vi "FTW-XML-Construct.vi"(5 "XML String":string, 11 "error in":errorcluster) -> (4 "XML Document":refnum<k20>, 15 "error out":errorcluster)   [LabVIEW 2013, in "XML.lvlib"]
uses:
  XML.lvlib
  DOMDefRefCommand.ctl
  <resource>/objmgr/DOMUserDefRef.rc
panel:
  # "Inputs"
  # "Outputs"
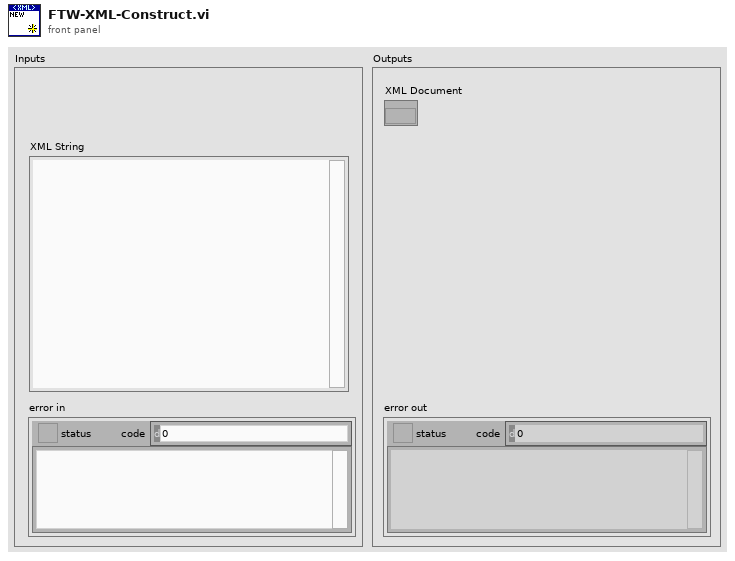
[diagram p1: front panel]
types:
  T1 = typedef "DOMDefRefCommand.ctl" = enum16{"No Command - Error", "Initialise", "Open Document", "Allocate RefNum", "Close Document"}
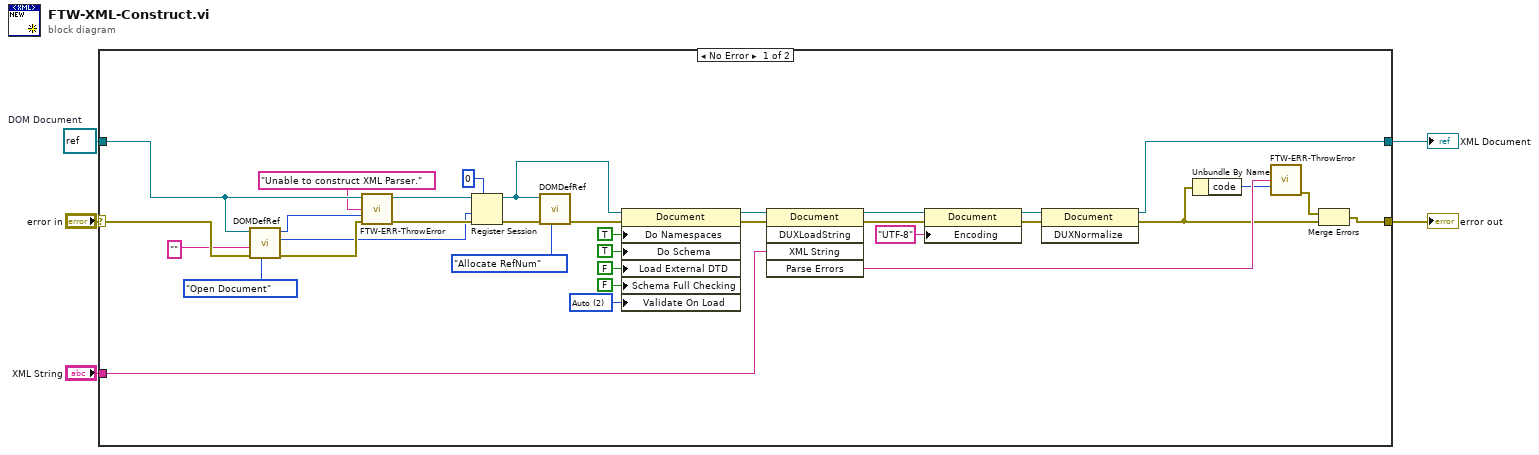
[diagram p0: block diagram]
diagram:
  w1 = refnum<k20> refnum  # DOM Document
  n1 = case shown="No Error" "error in" {
    selector: "error in" -> [w38 w40]
    tunnel: [w26 w40] -> w5
    tunnel: [w18 w39] -> w3
    tunnel: "XML String" -> [w30 _]
    tunnel: w1 -> [w25 w39]
    frame No Error {
      w33 = 2 items=["Never", "Always", "Auto"] ("Validate On Load")
      n2 = call "DOMDefRef.vi"("DOMUserDefRefCommand"=DOMDefRefCommand."Open Document", "error in (no error)"=w38, "Name"="", "Refnum in"=w25) -> ("error out"=w24:errorcluster, "Document Session"=w20:u64, "Return"=w21:i32)  [unwired: 2 in]
      n3 = call "FTW-ERR-ThrowError.vi"("Error Message"="Unable to construct XML Parser.", "Error Code"=w21, "error in"=w24) -> ("error out"=w23:errorcluster)  [unwired: 12 in]
      n4 = Register Session(7:0 ("cleanup mode (default to class = 0)"), 8:w23, 9:w20, 11:w25) -> (0:w9:errorcluster, 3:w8:refnum<k20>)  [unwired: 1 in]
      n5 = call "DOMDefRef.vi"("DOMUserDefRefCommand"=DOMDefRefCommand."Allocate RefNum", "error in (no error)"=w9, "Refnum in"=w8) -> ("error out"=w6:errorcluster)  [unwired: 3 in, 2 out]
      n6 = property class="Document"(reference=w8, error in=w6, "Do Namespaces"=TRUE ("Process Namespaces"), "Do Schema"=TRUE ("Process Schema"), "Load External DTD"=FALSE, "Schema Full Checking"=FALSE, "Validate On Load"=w33) -> (reference out=w31:refnum<k20>, error out=w32:errorcluster)
      n7 = invoke class="Document" method="DUXLoadString"(reference=w31, error in=w32, "XML String"=w30) -> (reference out=w16:refnum<k20>, error out=w15:errorcluster, "Parse Errors"=w29:string)  [unwired: 2 in, 2 out]
      n8 = property class="Document"(reference=w16, error in=w15, "Encoding"="UTF-8" ("Document Encoding")) -> (reference out=w14:refnum<k20>, error out=w13:errorcluster)
      n9 = invoke class="Document" method="DUXNormalize"(reference=w14, error in=w13) -> (reference out=w18:refnum<k20>, error out=w17:errorcluster)  [unwired: 1 in, 1 out]
      n10 = Unbundle By Name(w17) -> ("code"=w28:i32)
      n11 = call "FTW-ERR-ThrowError.vi"("Error Message"=w29, "Error Code"=w28) -> ("error out"=w27:errorcluster)  [unwired: 13 in]
      n12 = Merge Errors(w27, w17) -> (w26:errorcluster)
    }
    frame Error {
    }
  }
  "error out" <- w5
  "XML Document" <- w3
